vi "dev_det.vi"() -> (0 "DevDetect 2":u8)   [LabVIEW 2022 SP3]
uses:
  adcDLL_0001.dll
panel:
  in  "DevDetect":u8=4
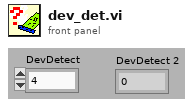
[diagram p1: front panel]
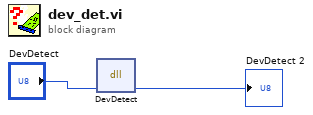
[diagram p0: block diagram]
diagram:
  n1 = dll-call lib="D:/LabVIEWSuite_64_OS/Spectrometers/ASEQ LR1/adcDLL_0001.dll" fn="DevDetect"("DevDetect"="DevDetect") -> ("DevDetect"=→"DevDetect 2":u8)  [unwired: 4 in, 2 out]
